vi "Alicat.vi"() -> ()   [LabVIEW 2018]
panel:
  in  "AR [ B-19200-COM8]":T1={" ID"="A", "Baud "=enum."19200", "VISA Sesssion In"="COM17"}
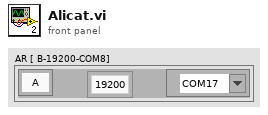
[diagram p1: front panel]
types:
  T1 = cluster{" ID":string, "Baud ":enum8{"2400", "9600", "19200", "38400", "57600", "115200", "Unknown"}, "VISA Sesssion In":refnum<visa-resource-name>}
  T2 = enum16{"open", "open or create", "create or replace", "create", "open (read-only)"}
  T3 = cluster{"Absolute Pressure":bool, "Gauge/Diff. Pressure":bool, "Barometric Pressure":bool, "Temperature":bool, "Volumetric":bool, "Mass":bool, "Setpoint":bool, "Valve Drive":bool, "Totalizer":bool, "Totalizer Timer":bool, "Totalizer Average Flow":bool, "Totalizer Peak Flow":bool, "Gas Selected":bool, "Tot. Timer Format":u16}
  T4 = cluster{"Abs. Pressure":string, "Gauge/Diff. Press.":string, "Barometric Press.":string, "Temperature":string, "Volume":string, "Mass":string, "Setpoint":string, "Valve Drive":string, "Totalizer":string, "Tot. Timer":string, "Tot. Avg. Flow":string, "Tot. Peak Flow":string}
  T5 = cluster{"Absolute Pressure":dbl, "Gauge/Diff. Pressure":dbl, "Barometric Pressure":dbl, "Temperature":dbl, "Volumetric Flow":dbl, "Mass Flow":dbl, "Setpoint":dbl, "Valve Drive":dbl, "Totalizer":dbl, "[hr]":dbl, "[min]":dbl, "[sec]":dbl, "Totalizer Average Flow":dbl, "Totalizer Peak Flow":dbl, "Gas selected":string}
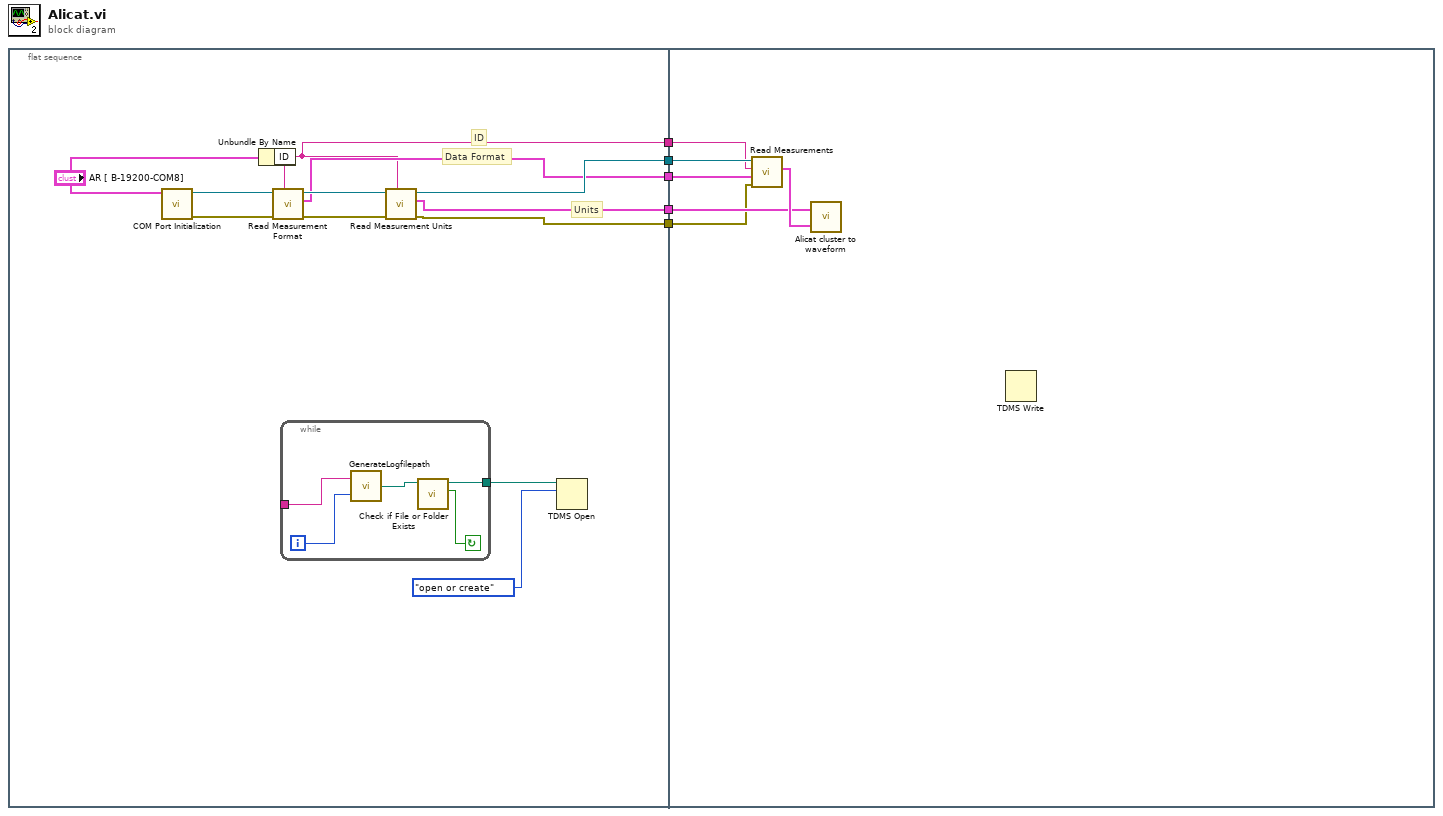
[diagram p0: block diagram]
diagram:
  n1 = flat-sequence {
    tunnel: [w12] -> w5
    tunnel: [w11] -> w4
    tunnel: [w10] -> w3
    tunnel: [w9] -> w2
    tunnel: [w8] -> w1
    tunnel: w5 -> [w27]
    tunnel: w4 -> [w26]
    tunnel: w3 -> [w25]
    tunnel: w2 -> [w24]
    tunnel: w1 -> [w23]
    frame #0 {
      # "Units"
      # "Data Format"
      # "ID"
      n2 = call "COM Port Initialization.vi"("Communication Settings"="AR [ B-19200-COM8]") -> ("error out"=w13:errorcluster, "VISA Session Out"=w14:refnum<visa-resource-name>)  [unwired: 9 in]
      n3 = Unbundle By Name("AR [ B-19200-COM8]") -> ("ID"=w9:string)
      n4 = call "Read Measurement Format.vi"("Unit ID (A)"=w9, "error in"=w13, "VISA Session In"=w14) -> ("error out"=w17:errorcluster, "Data Frame Format"=w10:T3, "VISA Session Out"=w16:refnum<visa-resource-name>)  [unwired: 6 in]
      n5 = while {
        tunnel: [w21] -> w7
        tunnel: _ -> [w18]
        i -> [w20]
        stop <- w22 continue-if-true
        n6 = call "GenerateLogfilepath.vi"("Number"=w20, "Instrument"=w18) -> ("Logfile Path"=w19:path)
        n7 = call <vilib>:"Check if File or Folder Exists.vi"("path"=w19) -> ("file or folder exists?"=w22:bool, "dup path"=w21:path)  [unwired: 8 in, 1 out]
      }
      n8 = call "Read Measurement Units.vi"("Unit ID (A)"=w9, "error in"=w17, "VISA Session In"=w16) -> ("error out"=w8:errorcluster, "Measurement Units"=w12:T4, "VISA Session Out"=w11:refnum<visa-resource-name>)  [unwired: 5 in, 1 out]
      n9 = TDMS Open(10:T2."open or create" ("operation (0:open)"), 11:w7) -> ()  [unwired: 5 in, 2 out]
    }
    frame #1 {
      n10 = call "Read Measurements.vi"("error in"=w23, "Data Frame Format In"=w25, "Unit ID (A)"=w24, "VISA Session In"=w26) -> ("Data Cluster"=w28:T5)  [unwired: 7 out]
      n11 = call "Alicat cluster to waveform.vi"("Data Cluster in"=w28, "Measurement Units in"=w27) -> ()  [unwired: 1 out]
      n12 = TDMS Write() -> ()  [unwired: 6 in, 4 out]
    }
  }
